vi "age364xa Single Channel Example no ovp.vi"(0 "VISA session":refnum<visa-resource-name>, 1 "Output Enabled (False)":bool, 5 "Voltage Level (0.0 Volts)":dbl format="%.2p", 7 "Current Limit (0 Amps)":dbl format="%.2p", 9 "OVP Limit (22.0 Volts)":dbl=22.0 format="%.2p", 11 "error in (no error)":errorcluster, 12 "OVP Enabled (True)":bool=TRUE) -> (4 "dup VISA session":refnum<visa-resource-name>, 15 "error out":errorcluster)   [LabVIEW 2012]
doc: "This VI configures the specifies power supply's channel to generate a DC voltage by taking the following steps:\n\n1) Configure current limit.\n\n2) Configure the over voltage protection.\n\n3) Configure the voltage level.\n\n4) Enable or disable the power output.\n\n5) Query the over voltage output state.\n\nNotes:\n\n(1) This VI takes a couple seconds to finish so that it may correctly get the current OVP value."
panel:
  # "For instructions,\nselect Show Context Help\nfrom the Help menu."
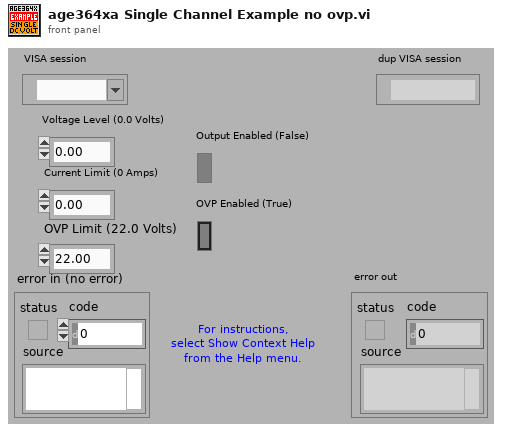
[diagram p1: front panel]
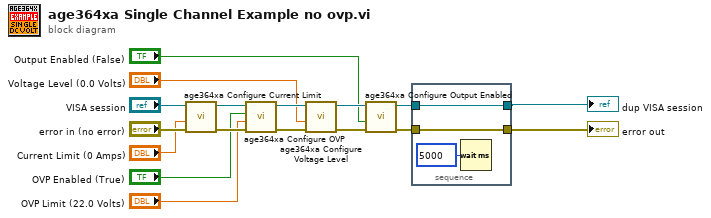
[diagram p0: block diagram]
diagram:
  n1 = call <instrlib>:"age364xa Configure Current Limit.vi"("error in (no error)"="error in (no error)", "Current Limit (0.0 Amps)"="Current Limit (0 Amps)", "VISA session"="VISA session") -> ("error out"=w17:errorcluster, "dup VISA session"=w16:refnum<visa-resource-name>)  [unwired: 7 in]
  n2 = call <instrlib>:"age364xa Configure OVP.vi"("error in (no error)"=w17, "Limit (22.0 Volts)"="OVP Limit (22.0 Volts)", "OVP Enabled (T: On)"="OVP Enabled (True)", "VISA session"=w16) -> ("error out"=w13:errorcluster, "dup VISA session"=w14:refnum<visa-resource-name>)  [unwired: 6 in]
  n3 = call <instrlib>:"age364xa Configure Voltage Level.vi"("error in (no error)"=w13, "Level (0.0 Volts)"="Voltage Level (0.0 Volts)", "VISA session"=w14) -> ("error out"=w10:errorcluster, "dup VISA session"=w11:refnum<visa-resource-name>)  [unwired: 7 in]
  n4 = call <instrlib>:"age364xa Configure Output Enabled.vi"("error in (no error)"=w10, "Output Enabled (F: Off)"="Output Enabled (False)", "VISA session"=w11) -> ("error out"=w6:errorcluster, "dup VISA session"=w7:refnum<visa-resource-name>)  [unwired: 7 in]
  n5 = stacked-sequence {
    tunnel: w7 -> [w19]
    tunnel: w6 -> [w18]
    tunnel: [w19] -> w2
    tunnel: [w18] -> w1
    frame #0 {
      n6 = Wait (ms)(milliseconds to wait=u32 5000) -> ()  [unwired: 1 out]
    }
  }
  "error out" <- w1
  "dup VISA session" <- w2
